vi "Centre image.vi"(8 "Stage Dimensions":T1={"X Dimension (pix)"=1000, "Y Dimension (pix)"=1000}, 9 "Image data":T2) -> (2 "Image Data":T2)   [LabVIEW 2018]
doc: "Positions the logo in the middle of the stage. This VI is used at the start."
uses:
  <vilib>/picture/picture.llb/imagedata.ctl
  Controls/Stage Dimensions (pix).ctl
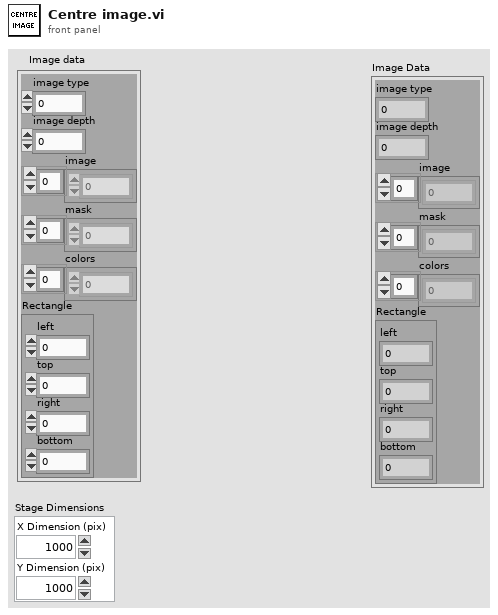
[diagram p1: front panel]
types:
  T1 = typedef "Stage Dimensions (pix).ctl" = cluster{"X Dimension (pix)":i16, "Y Dimension (pix)":i16}
  T2 = typedef "imagedata.ctl" = cluster{"image type":i32, "image depth":i32, "image":u8[], "mask":u8[], "colors":u32[], "Rectangle":cluster{"left":i16, "top":i16, "right":i16, "bottom":i16}}
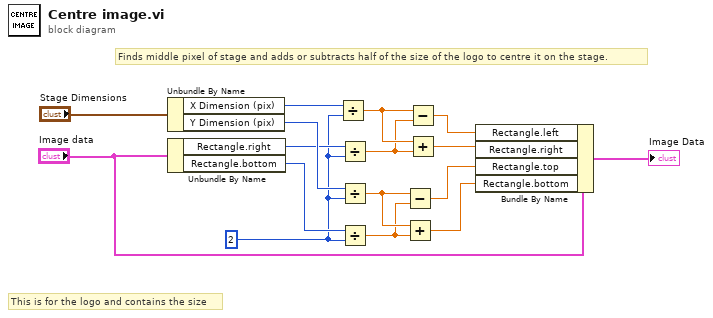
[diagram p0: block diagram]
diagram:
  w5 = i16 2 ("y")
  # "Finds middle pixel of stage and adds or subtracts half of the size of the logo to centre it on the stage."
  # "This is for the logo and contains the size"
  n1 = Unbundle By Name("Stage Dimensions") -> ("X Dimension (pix)"=w11:i16, "Y Dimension (pix)"=w10:i16)
  n2 = Unbundle By Name("Image data") -> ("Rectangle.right"=w7:i16, "Rectangle.bottom"=w6:i16)
  n3 = Divide(x=w11, y=w5) -> (x/y=w9:dbl)
  n4 = Divide(x=w7, y=w5) -> (x/y=w3:dbl)
  n5 = Divide(x=w10, y=w5) -> (x/y=w8:dbl)
  n6 = Divide(x=w6, y=w5) -> (x/y=w4:dbl)
  n7 = Subtract(x=w8, y=w4) -> (x-y=w1:dbl)
  n8 = Add(x=w8, y=w4) -> (x+y=w13:dbl)
  n9 = Subtract(x=w9, y=w3) -> (x-y=w15:dbl)
  n10 = Add(x=w9, y=w3) -> (x+y=w2:dbl)
  n11 = Bundle By Name(cluster="Image data", "Rectangle.left"=w15, "Rectangle.right"=w2, "Rectangle.top"=w1, "Rectangle.bottom"=w13) -> (→"Image Data":T2)
